vi "Create Template Properties.vi"(8 "error in (no error)":errorcluster, 11 "Acrobat Template in":refnum<class "Application.lvclass">) -> (0 "error out":errorcluster, 3 "Acrobat Template out":refnum<class "Application.lvclass">)   [LabVIEW 2017, in "Application.lvlib" / "Application.lvclass"]
uses:
  Application.lvclass
  Properties/App Properties.lvclass
  <vilib>/TSS/ACRObat Test Framework/Classes/Variable Engine/Class/Variable Engine.lvclass
  Properties/App Properties.lvclass/App Properties.ctl
  Application.lvclass/Application.ctl
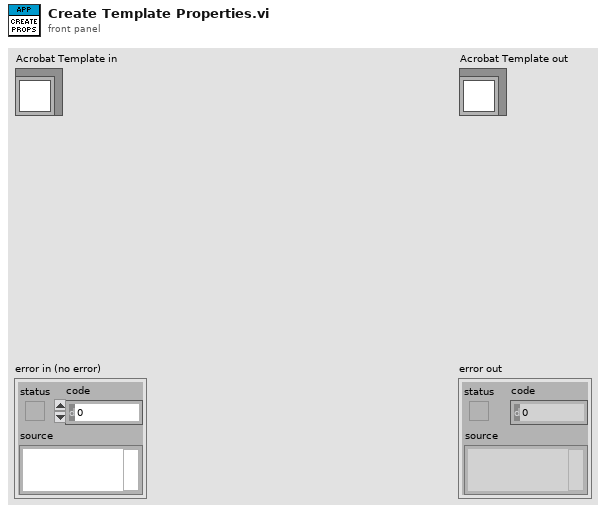
[diagram p1: front panel]
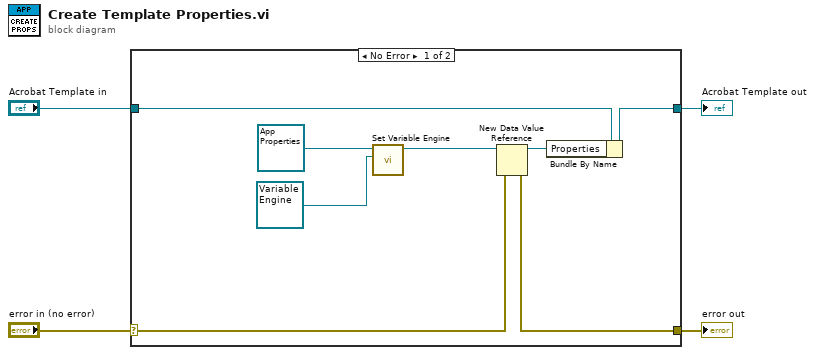
[diagram p0: block diagram]
diagram:
  n1 = case shown="No Error" "error in (no error)" {
    selector: "error in (no error)" -> [w10 w14]
    tunnel: [w9 w14] -> w3
    tunnel: [w11 w13] -> w1
    tunnel: "Acrobat Template in" -> [w12 w13]
    frame No Error {
      n2 = call "Set Variable Engine.vi"("Variable Engine"=refnum<class "Variable Engine.lvclass"> refnum, "App Properties in"=refnum<class "App Properties.lvclass"> refnum ("Acrobat Object Template.lvlib:Template Properties.lvclass")) -> ("App Properties out"=w6:refnum<class "App Properties.lvclass">)  [unwired: 8 in, 1 out]
      n3 = New Data Value Reference(data value=w6, error in=w10) -> (data value reference=w8:refnum<data-value>, error out=w9:errorcluster)
      n4 = Bundle By Name(cluster=w12, "Properties"=w8) -> (w11:refnum<class "Application.lvclass">)
    }
    frame Error {
    }
  }
  "error out" <- w3
  "Acrobat Template out" <- w1
